vi "test2.vi"() -> ()   [LabVIEW 2017]
panel:
  out "error out":errorcluster
  in  "error in (no error)":errorcluster
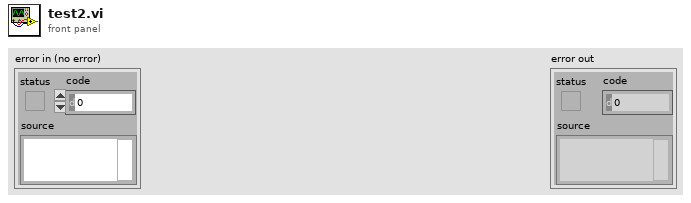
[diagram p1: front panel]
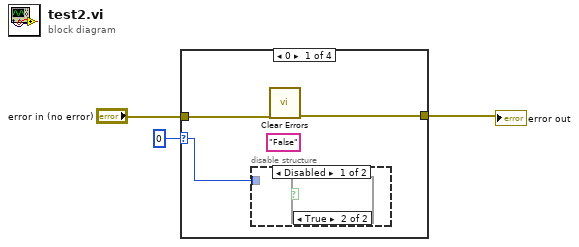
[diagram p0: block diagram]
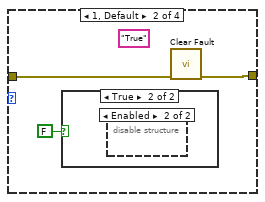
[diagram p4: hidden frame]
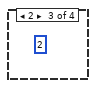
[diagram p7: hidden frame]
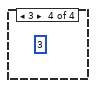
[diagram p8: hidden frame]
diagram:
  n1 = case shown="0" 0 {
    selector: 0 -> [w4 _ _ _]
    tunnel: "error in (no error)" -> [w6 w8 _ _]
    tunnel: [w5 w9 _ _] -> w2
    frame 0 {
      (unwired) "False"
      n2 = disable-structure shown="Disabled" {
        disable-tunnel: w4 -> [_ _]
        frame Disabled {
          n3 = case shown="True" {
            selector: _ -> [_ _]
            frame False {
            }
            frame True {
            }
          }
        }
        frame Enabled {
        }
      }
      n4 = call <vilib>:"Clear Errors.vi"("error in (no error)"=w6) -> ("error out"=w5:errorcluster)  [unwired: 5 in, 1 out]
    }
    frame 1, Default {
      (unwired) "True"
      n5 = case shown="True" FALSE {
        frame False {
        }
        frame True {
          n6 = disable-structure shown="Enabled" {
            frame Disabled {
            }
            frame Enabled {
            }
          }
        }
      }
      n7 = call <vilib>:"Clear Fault.vi"("error in (no error)"=w8) -> ("error out"=w9:errorcluster)  [unwired: 10 in]
    }
    frame 2 {
      (unwired) 2
    }
    frame 3 {
      (unwired) 3
    }
  }
  "error out" <- w2
